vi "Decimal to SNAFU.vi"(1 "Decimal Number":i64) -> (0 "SNAFU Number":string)   [LabVIEW 2020, in "AoC 2022.lvlib"]
uses:
  AoC 2022.lvlib
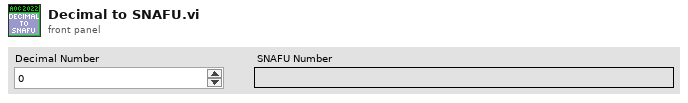
[diagram p1: front panel]
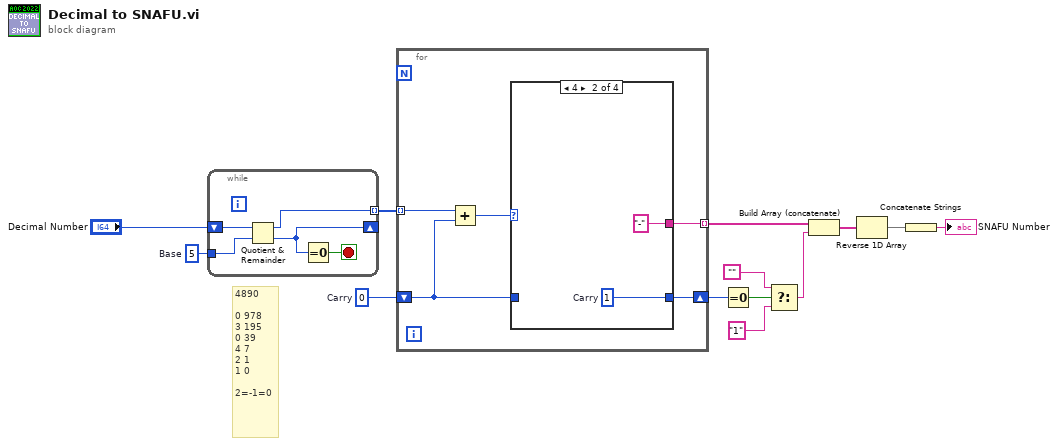
[diagram p0: block diagram]
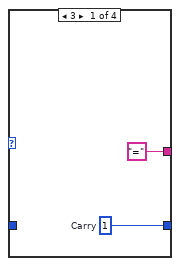
[diagram p2: hidden frame]
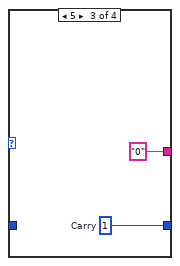
[diagram p3: hidden frame]
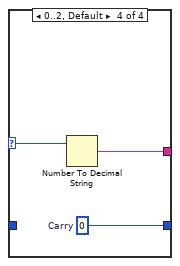
[diagram p4: hidden frame]
diagram:
  w4 = i64 0  # Carry
  w2 = i64 5  # Base
  # "4890\n\n0 978\n3 195\n0 39\n4 7\n2 1\n1 0\n\n2=-1=0"
  n1 = while {
    tunnel: w2 -> [w17]
    shift-right: [w14] -> _
    shift-left: "Decimal Number" -> [w18]
    tunnel: [w16] -> w3 mode=indexing
    stop <- w15 stop-if-true
    n2 = Quotient & Remainder(x=w18, y=w17) -> (x-y*floor(x/y)=w16:i64, floor(x/y)=w14:i64)
    n3 = Equal To 0?(x=w14) -> (x = 0?=w15:bool)
  }
  n4 = for {
    tunnel: w3 -> [w23] mode=indexing
    shift-right: [w21] -> w9
    shift-left: w4 -> [w20]
    tunnel: [w22] -> w5 mode=indexing
    n5 = Add(x=w23, y=w20) -> (x+y=w19:i64)
    n6 = case shown="4" w19 {
      selector: w19 -> [_ _ _ w30]
      tunnel: ["=" "-" "0" w32] -> w22
      tunnel: w20 -> [_ _ _ _]
      tunnel: [w25 w27 w29 w31] -> w21
      frame 3 {
        w25 = i64 1  # Carry
      }
      frame 4 {
        w27 = i64 1  # Carry
      }
      frame 5 {
        w29 = i64 1  # Carry
      }
      frame 0..2, Default {
        w31 = i64 0  # Carry
        n7 = Number To Decimal String(number=w30) -> (decimal integer string=w32:string)  [unwired: 1 in]
      }
    }
  }
  n8 = Equal To 0?(x=w9) -> (x = 0?=w8:bool)
  n9 = Select(t="", s=w8, f="1") -> (s? t:f=w13:string)
  n10 = Build Array (concatenate)(w5, w13) -> (w12:string[])
  n11 = Reverse 1D Array(array=w12) -> (reversed array=w6:string[])
  n12 = Concatenate Strings(w6) -> (→"SNAFU Number":string)
